vi "Generador_de_direcciones.vi"(10 "Numeric":i32, 11 "String":string) -> (3 "Path":path)   [LabVIEW 2016]
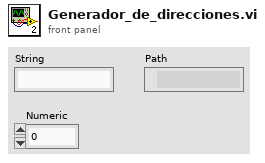
[diagram p1: front panel]
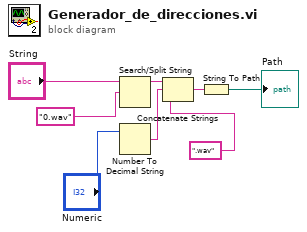
[diagram p0: block diagram]
diagram:
  n1 = Search/Split String(string="String", search string/char (-)="0.wav") -> (substring before match=w4:string)  [unwired: 1 in, 2 out]
  n2 = Number To Decimal String(number="Numeric") -> (decimal integer string=w5:string)  [unwired: 1 in]
  n3 = Concatenate Strings(w4, w5, ".wav") -> (w7:string)
  n4 = String To Path(string=w7) -> (path=→"Path":path)
